vi "AlliGator Set File Update LED.vi"(9 "error in (no error)":errorcluster, 10 "Off/On":bool) -> (1 "error out":errorcluster)   [LabVIEW 2021, in "AlliGator GUI.lvlib"]
doc: "Sets the status of the \"Dataset update needed\" LED."
uses:
  AlliGator GUI.lvlib
  AlliGator State Indicator.ctl
  AlliGator State Indicators List.ctl
  AlliGator Variables List.ctl
  AlliGator Globals, Variables & Constants.lvlib
  AlliGator Action Engine.lvlib
panel:
  out "State Indicators":T1
  # "see the AlliGator License on the block diagram (Ctrl+E or Window:Show Block Diagram)"
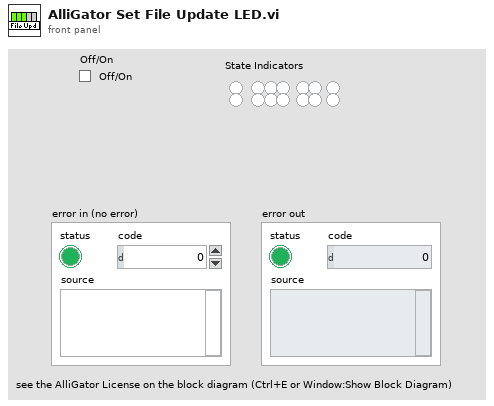
[diagram p1: front panel]
types:
  T1 = typedef "AlliGator GUI.lvlib/AlliGator State Indicator.ctl" = cluster{"Phasor Calibration Defined":bool, "Phasor Calibration Series Defined":bool, "Phasor Calibration Map Defined":bool, "Phasor Ratio Reference 1 Defined":bool, "Phasor Ratio Reference 2 Defined":bool, "Phasor Ratio Lifetime Reference 1 Defined ":bool, "Phasor Ratio Lifetime Reference 2 Defined":bool, "Phasor Calibration Used":bool, "Phasor Calibration Series Used":bool, "Phasor Calibration Map Used":bool, "Dataset Update Needed":bool, "Phasor Plot Update Needed":bool, "Reference/IRF Defined":bool, "Individual IRFs Defined":bool}
  T2 = typedef "AlliGator Action Engine.lvlib/AlliGator State Indicators List.ctl" = enum16{"Phasor Calibration Defined", "Phasor Calibration Series Defined", "Phasor Calibration Map Defined", "Phasor Reference 1 Defined", "Phasor Reference 2 Defined", "Lifetime Reference 1 Defined", "Lifetime Reference 2 Defined", "Phasor Calibration Used", "Phasor Calibration Series Used", "Phasor Calibration Map Used", "Dataset Update Needed", "Phasor Plot Update Needed", "Reference/IRF Defined", "Individual IRFs Defined"}
  T3 = typedef "AlliGator Globals, Variables & Constants.lvlib/AlliGator Variables List.ctl" = enum16{"---- GUI ----", "Initialization Status", "State Indicators Refnum", "Original AlliGator Menu Items", "Current Action Loop State", "Script in progress", "Playback", "Loop Playback", "Search ROI Used", "Search ROI", "Decay Graph Max Legend Size", "Intensity Graph Max Legend Size", "Decay Statistics Graph Max Legend Size", "Phasor Graph Max Legend Size", "Phasor Ratio Graph Max Legend Size", "Lifetime Graph Max Legend Size", "---- Files ----", "Export Dataset Frames as Individual Files", "Show Batch Export Help Balloons", "Frames in Dataset", "ptu File Frame Start Indices", "Current Frame in Dataset", "Current Frame Timestamp", "------ Python Plugins ------", "Python Plugins Information", "Python Session", "Valid Python Session?", "---- Source Image ----", "Dataset Loaded", "Dataset Metadata", "Dataset Channel", "Dataset Data Description", "Background Dataset Metadata", "Background Dataset Channel", "Background Dataset Data Description", "Background File Subtraction", "Background File Path", "Background File Pile-up Correction", "Background File Pixel Well Capacity", "Background File Scaling Factor", "Source Image ROIs", "Current Source Image ROI", "Source Image ROI Event Refnum", "X_Source Image Display Range", "X_Source Image Palette Information", "Source Image Palette List", "Source Image Scale", "Current Dataset Load Settings", "Source Image:ROI Overlay Color", "---- Image Profile Window ----", "Image Profile:Overlay ROI in Source Image", "Image Profile Window Event Refnum", "Image Profile:IntensityType", "Image Profile:Intensity Average Type", "Image Profile:Intensity-weighted SDV", "Image Profile:Box Profile Type", "Image Profile Window Open", "Image Profile:Plotted Fit Parameter", "X_Type of Displayed Image", "X_Time Gate Slider", "Dataset Path", "Source Image Overlay to Erase", "Is Displayed Image Accumulated", "White Light Image Modified", "Mask Image Modified", "Macrotime Gate Separation", "------ Phasor Graph -------", "Phasor Graph:Show Line", "---- Phasor Plot ---", "Phasor Plot Parameters Changed", "FLI Dataset Modified since last Phasor Plot Calculation", "Phasor Harmonics Data", "Selected Phasor Harmonics", "Phasor Harmonic Manager Event Refnum", "Phasor Plot ROIs", "Current Phasor Plot ROI", "Phasor Plot ROI Event Refnum", "Phasor Plot Image Reference Points", "Phasor Plot Computed", "Phasor Plot Palette Information", "Phasor Plot Palette List", "Phasor Ratio Palette Information", "Phasor Ratio Palette List", "Phasor Image Scale", "Phasor Plot Image Overlay to Erase", "Phasor Plot Image Elements to Update", "Current Phasor Plot Calculation Parameters", "Current Phasor Calibration Options", "Reset Cumulated Phasor Plot", "Phasor Ratio Reference 1", "Phasor Ratio Lifetime Reference 1", "Phasor Ratio Reference 1 Frequency", "Phasor Ratio Reference 2", "Phasor Ratio Lifetime Reference 2", "Phasor Ratio Reference 2 Frequency", "---- Decay Analysis ----", "Number of Selected Decays to Fit", "LS Fit Results", "LAR Fit Results", "BS Fit Results", "Last Decay Max - Min", "Best Fit Parameters", "Best Fit Parameter Names", "Actual Size X", "Actual Size Y", "Binning X", "Binning Y", "Actual # Gates", "Dataset Number", "Gates to...", "Gates Skipped", "Gates to keep", "Gate Step", "Gate Separation", "Reversed Gates", "Pile-up Correction", "Pixel Well Capacity", "Background Subtracted", "Background Subtraction Method", "Background Definition Range", "Background File (deprecated)", "Number of Dataset Accumulated", "Array of Accumulated Dataset Paths", "Do Averaged Datasets", "Destination File Path", "Process Plot Target", "Use 1/D as Phasor Frequency", "---- Decay Fit Parameter Map -----", "Decay Fit Parameter Map Palette Information", "Decay Fit Parameter Map Palette List", "Local Decay Graph Window Event Refnum", "------- Local Decay Window ---------", "Use normalized IRF for convolution", "----- Miscellaneous ----", "Skippable Dialog Windows Status"}
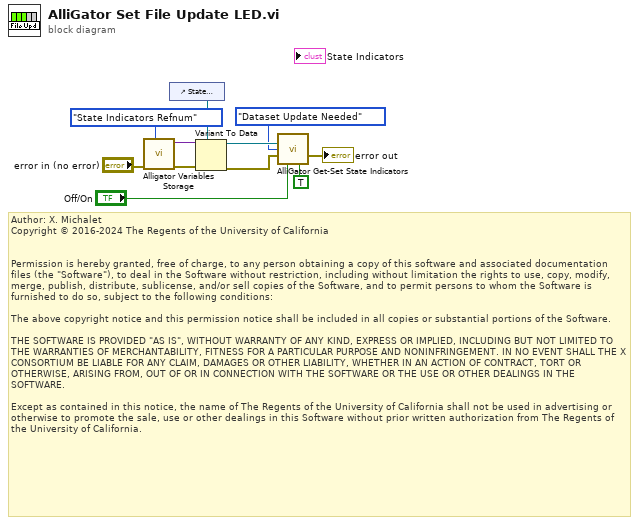
[diagram p0: block diagram]
diagram:
  # "Author: X. Michalet\nCopyright © 2016-2024 The Regents of the University of California\n \n\nPermission is hereby granted, free of charge, to any person obtaining a copy of this software and associated documentation files (the \"Software\"), to deal in the Software without restriction, including without limitation the rights to use, copy, modify, merge, publish, distribute, sublicense, and/or sell copies of the Software, and to permit persons to whom the Software is furnished to do so, subject to the following conditions:\n\nThe above copyright notice and this permission notice shall be included in all copies or substantial portions of the Software.\n\nTHE SOFTWARE IS PROVIDED \"AS IS\", WITHOUT WARRANTY OF ANY KIND, EXPRESS OR IMPLIED, INCLUDING BUT NOT LIMITED TO THE WARRANTIES OF MERCHANTABILITY, FITNESS FOR A PARTICULAR PURPOSE AND NONINFRINGEMENT. IN NO EVENT SHALL THE X CONSORTIUM BE LIABLE FOR ANY CLAIM, DAMAGES OR OTHER LIABILITY, WHETHER IN AN ACTION OF CONTRACT, TORT OR OTHERWISE, ARISING FROM, OUT OF OR IN CONNECTION WITH THE SOFTWARE OR THE USE OR OTHER DEALINGS IN THE SOFTWARE.\n\nExcept as contained in this notice, the name of The Regents of the University of California shall not be used in advertising or otherwise to promote the sale, use or other dealings in this Software without prior written authorization from The Regents of the University of California."
  n1 = call "Alligator Variables Storage.vi"("AlliGator Variable"=AlliGator_Variables_List."State Indicators Refnum" ("Alligator Variable"), "Error In"="error in (no error)") -> ("Error Out"=w9:errorcluster, "Data out"=w10:variant)  [unwired: 7 in, 1 out]
  n2 = control-ref of="State Indicators"() -> (w8:refnum<vi>)
  n3 = Variant To Data(error in=w9, type=w8, Variant=w10) -> (data=w7:refnum<vi>, error out=w6:errorcluster)
  n4 = call "AlliGator Get-Set State Indicators.vi"("State Indicators Refnum"=w7, "AlliGator State Indicators List"=AlliGator_State_Indicators_List."Dataset Update Needed", "Error In"=w6, "ON/OFF"="Off/On", "Set (T)/Get"=TRUE) -> ("Error Out"=→"error out":errorcluster)  [unwired: 8 in, 2 out]
